vi "endEventToStringArray.vi"(8 "error in (no error)":errorcluster, 11 "RampDown in":refnum<class "RampDown.lvclass">) -> (0 "error out":errorcluster, 2 "eventStringArray":string[](array[string]), 3 "RampDown out":refnum<class "RampDown.lvclass">)   [LabVIEW 2011, in "Tools.lvlib" / "Scripting.lvlib" / "RampDown.lvclass"]
uses:
  RampDown.lvclass
  ScriptEvent.lvclass
  RampEvent/RampEvent.lvclass
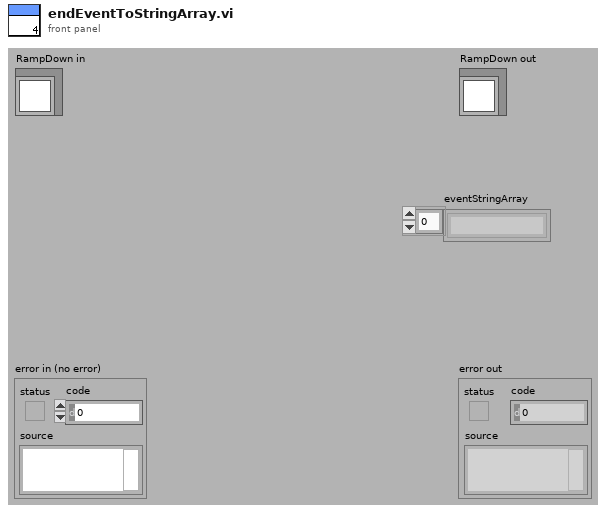
[diagram p1: front panel]
types:
  T1 = cluster{"rampTime":dbl, "timeStep":dbl, "dataValueStep":dbl}
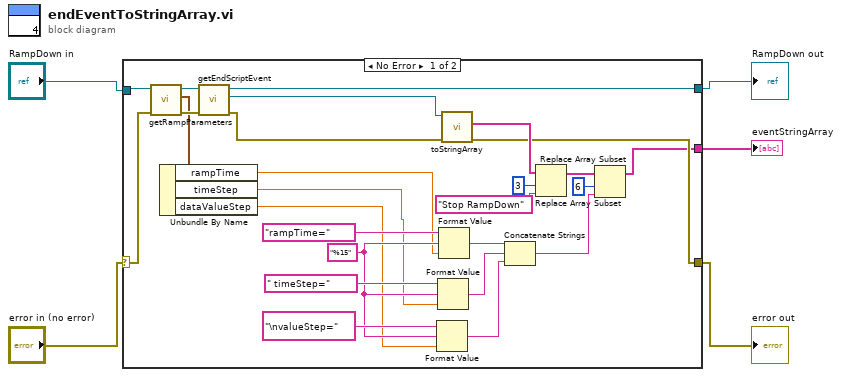
[diagram p0: block diagram]
diagram:
  n1 = case shown="No Error" "error in (no error)" {
    selector: "error in (no error)" -> [w15 w32]
    tunnel: [w7 w33] -> w2
    tunnel: "RampDown in" -> [w6 w33]
    tunnel: [w18 w32] -> w3
    tunnel: [w17 _] -> w1
    frame No Error {
      w28 = "%15"
      n2 = call "getRampParameters.vi"("error in (no error)"=w15, "RampEvent in"=w6) -> ("error out"=w13:errorcluster, "RampParameters"=w12:T1, "RampEvent out"=w16:refnum<class "RampDown.lvclass">)  [unwired: 7 in]
      n3 = Unbundle By Name(w12) -> ("rampTime"=w11:dbl, "timeStep"=w10:dbl, "dataValueStep"=w9:dbl)
      n4 = call "getEndScriptEvent.vi"("error in (no error)"=w13, "RampEvent.lvclass in"=w16) -> ("error out"=w14:errorcluster, "ScriptEvent.lvclass"=w8:refnum<class "ScriptEvent.lvclass">, "RampEvent.lvclass out"=w7:refnum<class "RampDown.lvclass">)  [unwired: 7 in]
      n5 = Format Value(string ("")="\nvalueStep=", format string=w28, value (0)=w9) -> (output string=w21:string)
      n6 = Format Value(string ("")=" timeStep=", format string=w28, value (0)=w10) -> (output string=w22:string)
      n7 = Format Value(string ("")="rampTime=", format string=w28, value (0)=w11) -> (output string=w23:string)
      n8 = call-dynamic "toStringArray.vi"("error in (no error)"=w14, "ScriptEvent in"=w8) -> ("error out"=w18:errorcluster, "eventStringArray"=w19:string[])  [unwired: 7 in, 1 out]
      n9 = Concatenate Strings(w23, w22, w21) -> (w20:string)
      n10 = Replace Array Subset(array=w19, new element="Stop RampDown", index=3) -> (w26:string[])
      n11 = Replace Array Subset(array=w26, new element=w20, index=6) -> (w17:string[])
    }
    frame Error {
    }
  }
  "error out" <- w3
  "RampDown out" <- w2
  "eventStringArray" <- w1
